vi "QTrkQueueFrame.vi"(0 "QTrk Instance":T2, 1 "frame#":u32, 2 "Clear first 4 bytes in frame? (F)":bool, 3 "timestamp":u32, 5 "error in (no error)":errorcluster, 6 "Image":T1, 7 "ROI Positions (corner-based)":cluster{"X":i32, "Y":i32}[](array[cluster]), 8 "ZLUT Index offset (0)":i32) -> (14 "QTrk Instance (out)":T2, 15 "timestamp from frame":u32, 19 "error out":errorcluster)   [LabVIEW 2011]
uses:
  QTrkInstance.ctl
  <vilib>/vision/Image Controls.llb/IMAQ Image.ctl
  QTrkLocalizationJob.ctl
  XYZf.ctl
  QTrkPixelDataType.ctl
  QTrkDLL.vi
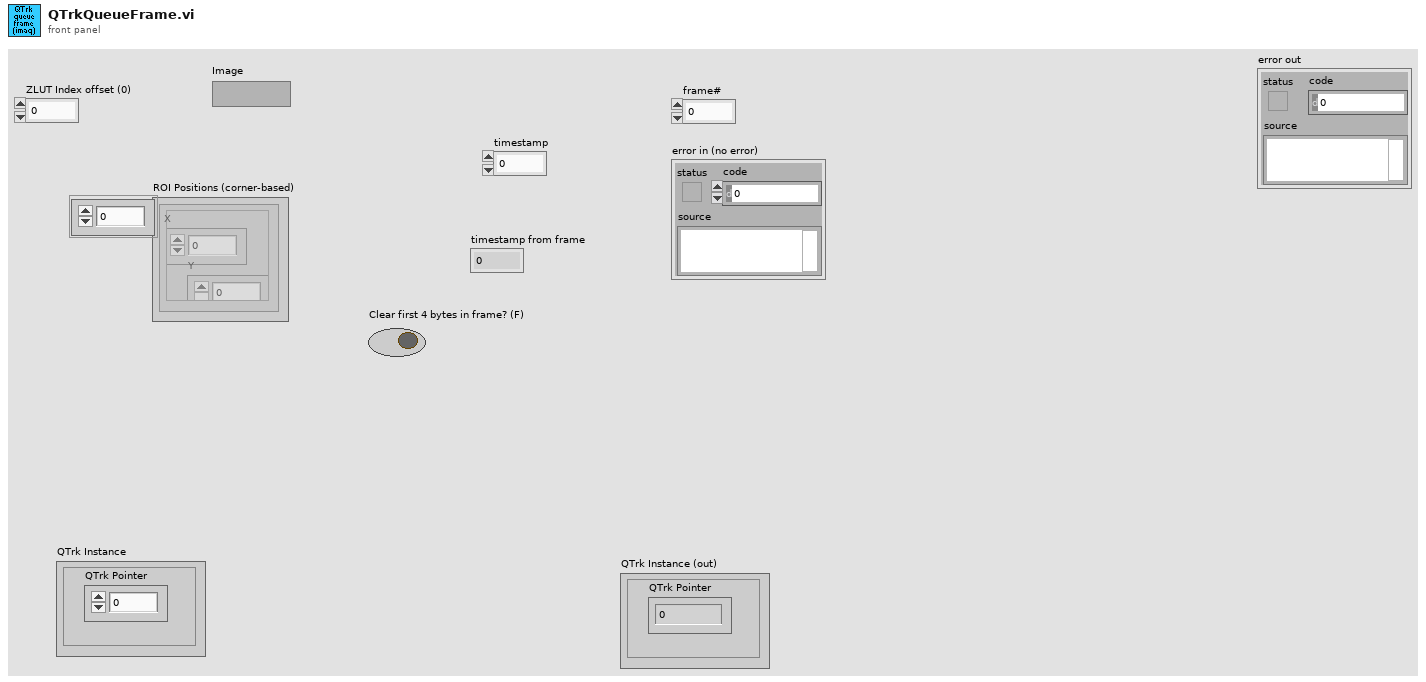
[diagram p1: front panel]
types:
  T1 = typedef "IMAQ Image.ctl" = refnum<image>
  T2 = typedef "QTrkInstance.ctl" = cluster{"QTrk Pointer":u64}
  T3 = typedef "QTrkLocalizationJob.ctl" = cluster{"Frame#":u32, "Timestamp":u32, "ZLUT Index / bead#":i32, "Initial guess":T4}
  T4 = typedef "XYZf.ctl" = cluster{"X":sgl, "Y":sgl, "Z":sgl}
  T5 = enum32{"Map Pixel Pointer", "Unmap Pixel Pointer", "Get Pixels Infos"}
  T6 = typedef "QTrkPixelDataType.ctl" = enum16{"QTrkU8", "QTrkU16", "QTrkFloat"}
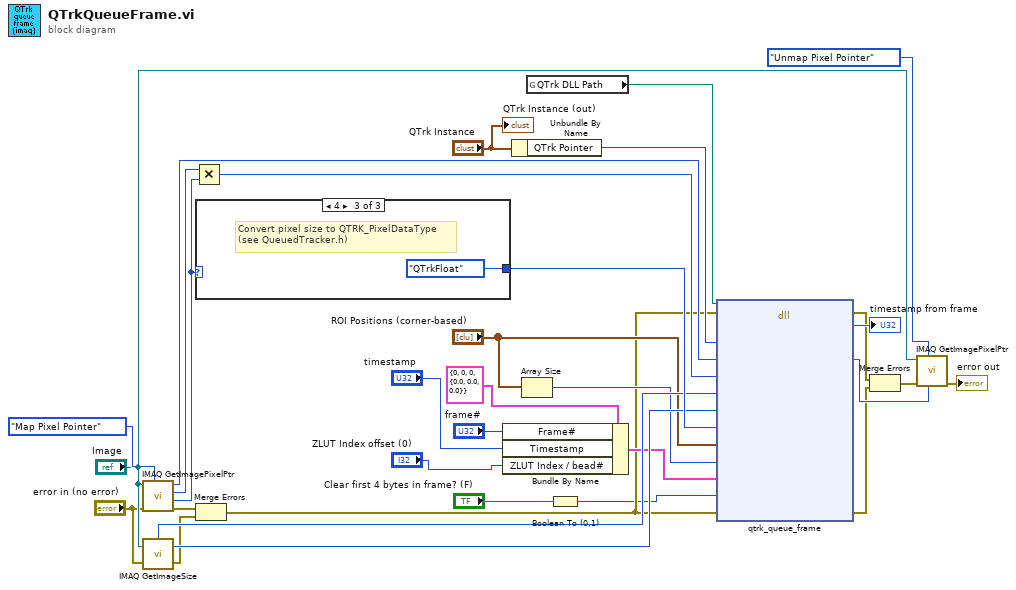
[diagram p0: block diagram]
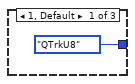
[diagram p2: hidden frame]
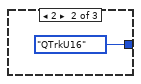
[diagram p3: hidden frame]
diagram:
  n1 = call "IMAQ GetImagePixelPtr"("Function"=T5."Map Pixel Pointer", "error in (no error)"="error in (no error)", "Image"="Image") -> ("error out"=w16:errorcluster, "Pixel Size (Bytes)"=w24:i32, "LineWidth(Pixels)"=w25:i32, "Pixel Pointer out"=w26:u64)  [unwired: 3 in, 2 out]
  n2 = call "IMAQ GetImageSize"("Image"="Image", "error in (no error)"="error in (no error)") -> ("Y Resolution"=w20:i32, "X Resolution"=w21:i32, "error out"=w17:errorcluster)  [unwired: 2 in]
  n3 = Multiply(x=w25, y=w24) -> (x*y=w22:i32)
  n4 = case shown="4" w24 {
    tunnel: [QTrkPixelDataType."QTrkU8" ("Pixel data type") QTrkPixelDataType."QTrkU16" ("Pixel data type") QTrkPixelDataType."QTrkFloat" ("Pixel data type")] -> w23
    frame 1, Default {
    }
    frame 2 {
    }
    frame 4 {
      # "Convert pixel size to QTRK_PixelDataType\n(see QueuedTracker.h)"
    }
  }
  n5 = Merge Errors(w16, w17) -> (w4:errorcluster)
  n6 = Bundle By Name(cluster=T3 {"Frame#"=0, "Timestamp"=0, "ZLUT Index / bead#"=0, "Initial guess"={"X"=0.0, "Y"=0.0, "Z"=0.0}} ("Queue Params"), "Frame#"="frame#", "Timestamp"="timestamp", "ZLUT Index / bead#"="ZLUT Index offset (0)") -> (w9:T3)
  n7 = Unbundle By Name("QTrk Instance") -> ("QTrk Pointer"=w28:u64)
  n8 = Array Size(array="ROI Positions (corner-based)") -> (size(s)=w14:i32)
  n9 = global read "QTrkDLL.vi" "QTrk DLL Path"() -> (w27:path)
  n10 = Boolean To (0,1)(Boolean="Clear first 4 bytes in frame? (F)") -> (0, 1=w1:i16)
  n11 = dll-call lib="D:/jcnossen1/cudaqi-tracker/bin/jtrk-labview.dll" fn="qtrk_queue_frame"(path in=w27, error in=w4, "tracker"=w28, "image"=w26, "pitch"=w22, "width"=w21, "height"=w20, "bytesPerPixel"=w23, "positions"="ROI Positions (corner-based)", "numROI"=w14, "jobInfo"=w9, "flags"=w1, "err"=w4) -> (error out=w6:errorcluster, "timestamp from frame"=→"timestamp from frame":u32, "image"=w19:u64, "err"=w3:errorcluster)  [unwired: 10 in, 1 out]
  n12 = Merge Errors(w6, w3) -> (w5:errorcluster)
  n13 = call "IMAQ GetImagePixelPtr"("Pixel Pointer in"=w19, "Function"=T5."Unmap Pixel Pointer", "error in (no error)"=w5, "Image"="Image") -> ("error out"=→"error out":errorcluster)  [unwired: 2 in, 5 out]
  "QTrk Instance (out)" <- "QTrk Instance"
